vi "Init.vi"(8 "error in":errorcluster, 11 "CFG Base in":refnum<class "EL Control Load CFG.lvclass">) -> (0 "error out":errorcluster, 3 "CFG Base out":refnum<class "EL Control Load CFG.lvclass">)   [LabVIEW 2023, in "EL Control Load CFG.lvclass"]
uses:
  EL Control Load CFG.lvclass
  SCPI PE Input.ctl
  EL Control Load CFG.lvclass/EL Control Load CFG.ctl
  <vilib>/Instr/_visa.llb/VISA Configure Serial Port (Instr).vi
  Configuration/Configuration Semaphore/CFG Semaphore.lvclass
panel:
  out "Instr Info":variant
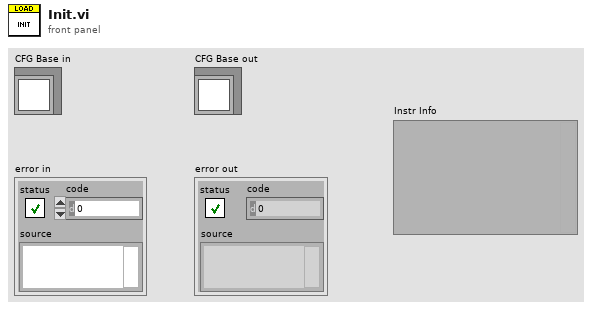
[diagram p1: front panel]
types:
  T1 = typedef "SCPI PE Input.ctl" = cluster{"Action":enum16{"Write", "Query"}, "SCPI":string}
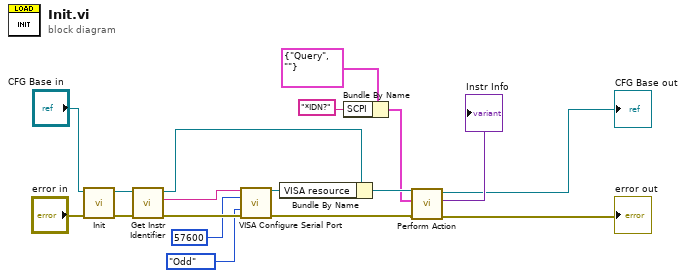
[diagram p0: block diagram]
diagram:
  n1 = call-parent "Init.vi"("error in"="error in", "CFG Base in"="CFG Base in") -> ("error out"=w18:errorcluster, "CFG Base out"=w15:refnum<class "EL Control Load CFG.lvclass">)  [unwired: 8 in]
  n2 = call-dynamic "Get Instr Identifier.vi"("error in (no error)"=w18, "Configuration Base in"=w15) -> ("error out"=w14:errorcluster, "Instr Ident"=w13:string, "Configuration Base out"=w10:refnum<class "EL Control Load CFG.lvclass">)  [unwired: 7 in]
  n3 = call-poly "VISA Configure Serial Port"("VISA resource name"=w13, "baud rate (9600)"=u32 57600, "parity (0:none)"=enum16{"None", "Odd", "Even", "Mark", "Space"}."Odd", "error in (no error)"=w14) -> ("VISA resource name out"=w7:refnum<visa-resource-name>, "error out"=w9:errorcluster)  [unwired: 6 in, 4 out]
  n4 = Bundle By Name(cluster=w10, "VISA resource"=w7) -> (w6:refnum<class "EL Control Load CFG.lvclass">)
  n5 = Bundle By Name(cluster=T1 {"Action"=enum."Query", "SCPI"=""} ("PE Input"), "SCPI"="*IDN?") -> (w3:T1)
  n6 = call-dynamic "Perform Action.vi"("error in"=w9, "Input"=w3, "Control Load CFG in"=w6) -> ("error out"=→"error out":errorcluster, "Output"=→"Instr Info":variant, "Control Load CFG out"=→"CFG Base out":refnum<class "EL Control Load CFG.lvclass">)  [unwired: 6 in]
